vi "getAdditionalDataXML.vi"(8 "error in (no error)":errorcluster, 11 "SingleToneRamp in":refnum<class "SingleToneRamp.lvclass">) -> (0 "error out":errorcluster, 2 "additionalDataXML":refnum<class "xmlNode.lvclass">, 3 "SingleToneRamp out":refnum<class "SingleToneRamp.lvclass">)   [LabVIEW 2009, in "Tools.lvlib" / "Scripting.lvlib" / "SingleToneRamp.lvclass"]
uses:
  SingleToneRamp.lvclass
  xmlNode/xmlNode.lvclass
  SingleToneRamp.lvclass/SingleToneRamp.ctl
  ScriptEvent.lvclass
  SingleTone.lvclass
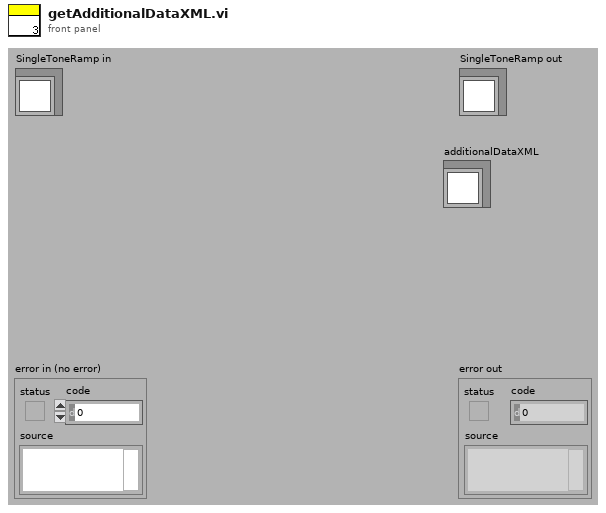
[diagram p1: front panel]
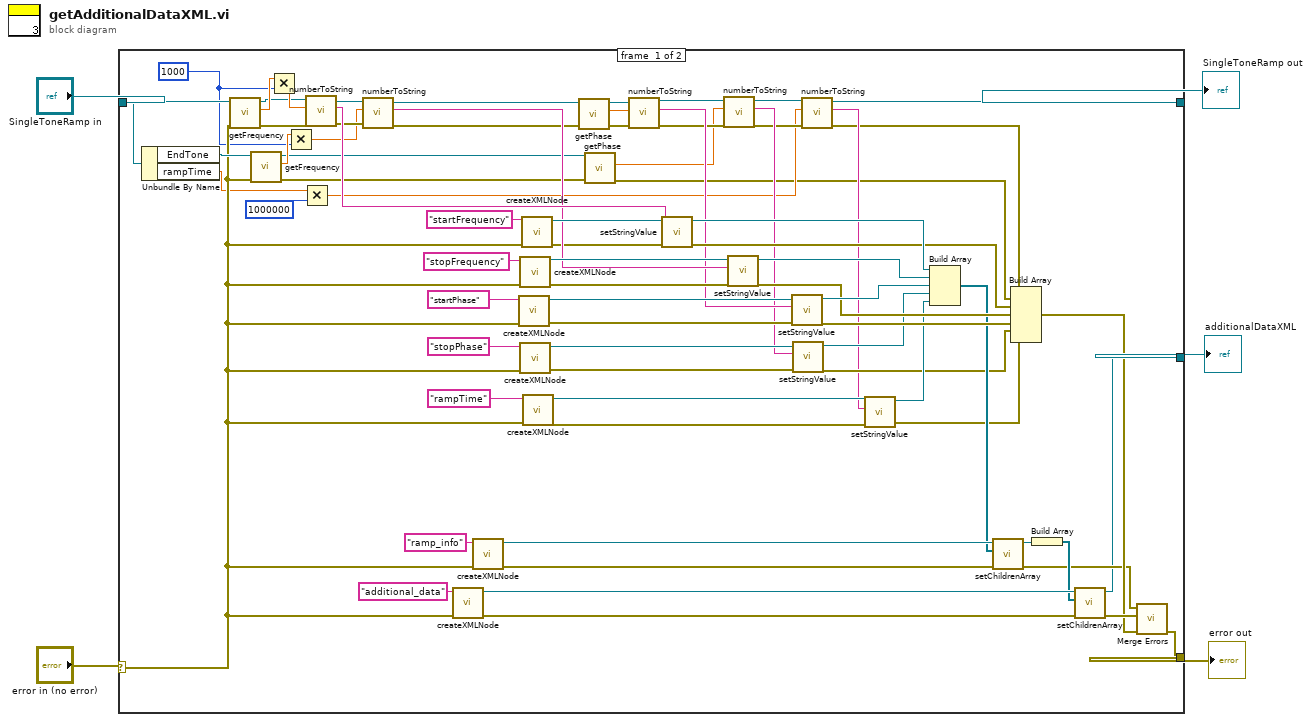
[diagram p0: block diagram]
diagram:
  n1 = case shown="No Error" "error in (no error)" {
    selector: "error in (no error)" -> [w31 w80]
    tunnel: "SingleToneRamp in" -> [w34 w81]
    tunnel: [w9 w81] -> w4
    tunnel: [w55 w80] -> w1
    tunnel: [w54 _] -> w2
    frame #0 {
      w26 = 1000
      n2 = Unbundle By Name(w34) -> ("EndTone"=w32:refnum<class "SingleTone.lvclass">, "rampTime"=w14:dbl)
      n3 = call "getFrequency.vi"("error in (no error)"=w31, "SingleTone.lvclass in"=w34) -> ("error out"=w28:errorcluster, "frequency"=w33:dbl, "SingleTone.lvclass out"=w29:refnum<class "SingleToneRamp.lvclass">)  [unwired: 7 in]
      n4 = call "getFrequency.vi"("error in (no error)"=w31, "SingleTone.lvclass in"=w32) -> ("error out"=w19:errorcluster, "frequency"=w30:dbl, "SingleTone.lvclass out"=w20:refnum<class "SingleTone.lvclass">)  [unwired: 7 in]
      n5 = Multiply(x=w33, y=w26) -> (x*y=w51:dbl)
      n6 = Multiply(x=w30, y=w26) -> (x*y=w27:dbl)
      n7 = Multiply(x=w14, y=1000000) -> (x*y=w10:dbl)
      n8 = call "numberToString.vi"("error in (no error)"=w28, "Numeric"=w51, "ScriptEvent in"=w29) -> ("error out"=w46:errorcluster, "String"=w50:string, "ScriptEvent out"=w49:refnum<class "SingleToneRamp.lvclass">)  [unwired: 6 in]
      n9 = call "numberToString.vi"("error in (no error)"=w46, "Numeric"=w27, "ScriptEvent in"=w49) -> ("error out"=w24:errorcluster, "String"=w48:string, "ScriptEvent out"=w25:refnum<class "SingleToneRamp.lvclass">)  [unwired: 6 in]
      n10 = call "createXMLNode.vi"("error in (no error)"=w31, "name"="additional_data") -> ("error out"=w52:errorcluster, "xmlNode out"=w61:refnum<class "xmlNode.lvclass">)  [unwired: 8 in]
      n11 = call "createXMLNode.vi"("error in (no error)"=w31, "name"="ramp_info") -> ("error out"=w62:errorcluster, "xmlNode out"=w64:refnum<class "xmlNode.lvclass">)  [unwired: 8 in]
      n12 = call "createXMLNode.vi"("error in (no error)"=w31, "name"="startPhase") -> ("error out"=w71:errorcluster, "xmlNode out"=w72:refnum<class "xmlNode.lvclass">)  [unwired: 8 in]
      n13 = call "createXMLNode.vi"("error in (no error)"=w31, "name"="stopFrequency") -> ("error out"=w73:errorcluster, "xmlNode out"=w74:refnum<class "xmlNode.lvclass">)  [unwired: 8 in]
      n14 = call "createXMLNode.vi"("error in (no error)"=w31, "name"="stopPhase") -> ("error out"=w42:errorcluster, "xmlNode out"=w43:refnum<class "xmlNode.lvclass">)  [unwired: 8 in]
      n15 = call "createXMLNode.vi"("error in (no error)"=w31, "name"="startFrequency") -> ("error out"=w45:errorcluster, "xmlNode out"=w75:refnum<class "xmlNode.lvclass">)  [unwired: 8 in]
      n16 = call "createXMLNode.vi"("error in (no error)"=w31, "name"="rampTime") -> ("error out"=w38:errorcluster, "xmlNode out"=w39:refnum<class "xmlNode.lvclass">)  [unwired: 8 in]
      n17 = call "getPhase.vi"("error in (no error)"=w24, "SingleTone.lvclass in"=w25) -> ("error out"=w22:errorcluster, "phase"=w21:dbl, "SingleTone.lvclass out"=w23:refnum<class "SingleToneRamp.lvclass">)  [unwired: 7 in]
      n18 = call "getPhase.vi"("error in (no error)"=w19, "SingleTone.lvclass in"=w20) -> ("error out"=w7:errorcluster, "phase"=w16:dbl)  [unwired: 7 in, 1 out]
      n19 = call "numberToString.vi"("error in (no error)"=w22, "Numeric"=w21, "ScriptEvent in"=w23) -> ("error out"=w17:errorcluster, "String"=w47:string, "ScriptEvent out"=w18:refnum<class "SingleToneRamp.lvclass">)  [unwired: 6 in]
      n20 = call-dynamic "setStringValue.vi"("error in (no error)"=w45, "stringValue"=w50, "xmlNode.lvclass in"=w75) -> ("error out"=w67:errorcluster, "xmlNode.lvclass out"=w70:refnum<class "xmlNode.lvclass">)  [unwired: 7 in]
      n21 = call "numberToString.vi"("error in (no error)"=w17, "Numeric"=w16, "ScriptEvent in"=w18) -> ("error out"=w11:errorcluster, "String"=w15:string, "ScriptEvent out"=w12:refnum<class "SingleToneRamp.lvclass">)  [unwired: 6 in]
      n22 = call-dynamic "setStringValue.vi"("error in (no error)"=w73, "stringValue"=w48, "xmlNode.lvclass in"=w74) -> ("error out"=w66:errorcluster, "xmlNode.lvclass out"=w69:refnum<class "xmlNode.lvclass">)  [unwired: 7 in]
      n23 = call-dynamic "setStringValue.vi"("error in (no error)"=w71, "stringValue"=w47, "xmlNode.lvclass in"=w72) -> ("error out"=w65:errorcluster, "xmlNode.lvclass out"=w68:refnum<class "xmlNode.lvclass">)  [unwired: 7 in]
      n24 = call-dynamic "setStringValue.vi"("error in (no error)"=w42, "stringValue"=w15, "xmlNode.lvclass in"=w43) -> ("error out"=w36:errorcluster, "xmlNode.lvclass out"=w41:refnum<class "xmlNode.lvclass">)  [unwired: 7 in]
      n25 = call "numberToString.vi"("error in (no error)"=w11, "Numeric"=w10, "ScriptEvent in"=w12) -> ("error out"=w6:errorcluster, "String"=w8:string, "ScriptEvent out"=w9:refnum<class "SingleToneRamp.lvclass">)  [unwired: 6 in]
      n26 = call-dynamic "setStringValue.vi"("error in (no error)"=w38, "stringValue"=w8, "xmlNode.lvclass in"=w39) -> ("error out"=w35:errorcluster, "xmlNode.lvclass out"=w37:refnum<class "xmlNode.lvclass">)  [unwired: 7 in]
      n27 = Build Array(w70, w69, w68, w41, w37) -> (w63:refnum<class "xmlNode.lvclass">[])
      n28 = call-dynamic "setChildrenArray.vi"("error in (no error)"=w62, "Children"=w63, "xmlNode.lvclass in"=w64) -> ("error out"=w56:errorcluster, "xmlNode.lvclass out"=w60:refnum<class "xmlNode.lvclass">)  [unwired: 7 in]
      n29 = Build Array(w6, w7, w67, w66, w65, w36, w35) -> (w57:errorcluster[])
      n30 = Build Array(w60) -> (w59:refnum<class "xmlNode.lvclass">[])
      n31 = call-dynamic "setChildrenArray.vi"("error in (no error)"=w52, "Children"=w59, "xmlNode.lvclass in"=w61) -> ("error out"=w58:errorcluster, "xmlNode.lvclass out"=w54:refnum<class "xmlNode.lvclass">)  [unwired: 7 in]
      n32 = call <vilib>:"Merge Errors.vi"("error array in"=w57, "error in 2 (no error)"=w58, "error in 1 (no error)"=w56) -> ("error out"=w55:errorcluster)  [unwired: 4 in]
    }
    frame #1 {
    }
  }
  "error out" <- w1
  "SingleToneRamp out" <- w4
  "additionalDataXML" <- w2
